vi "BinaryADR112Voltmeter.vi"() -> ()   [LabVIEW 2017]
doc: "This vi interfaces with the ADR 112 Serial Board and acts as a voltmeter, displaying the voltage as a graphical needle guage as well as a binary led array."
uses:
  <vilib>/Instr/_visa.llb/VISA Configure Serial Port (Instr).vi
panel:
  in  "Channel":i32
  in  "COM":refnum<visa-resource-name>
  in  "On":bool
  out "Voltmeter":dbl(knob) scale=0.0..5.0
  out "12 Bit Binary Display":bool[](array[boolean])
  # "Most Significant Bit"
  # "Least Significant Bit"
  # "V"
  # "Off"
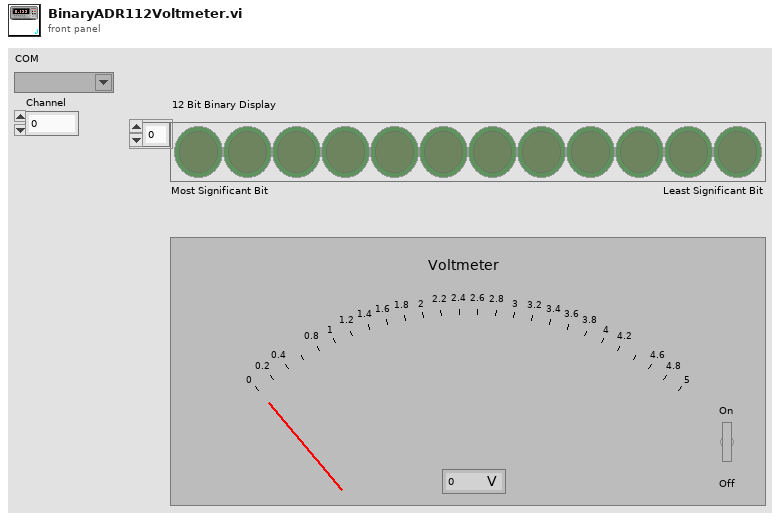
[diagram p1: front panel]
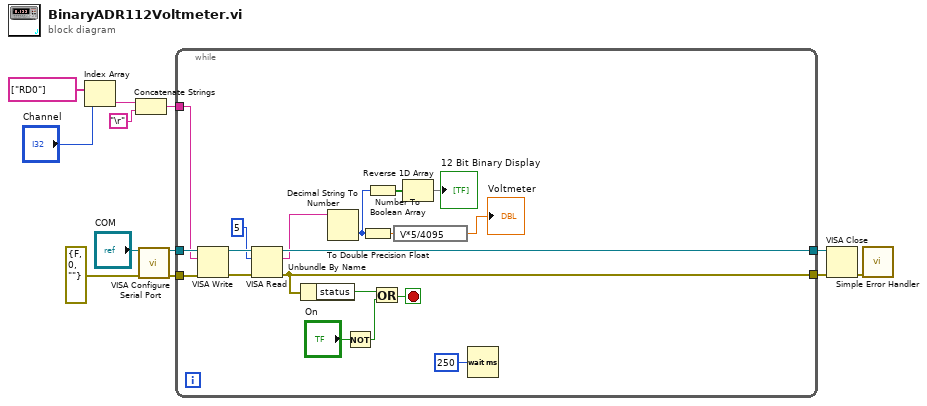
[diagram p0: block diagram]
diagram:
  n1 = Index Array(array=string[] ["RD0"], index="Channel") -> (element=w6:string)
  n2 = Concatenate Strings(w6, "\r") -> (w4:string)
  n3 = call-poly "VISA Configure Serial Port"("VISA resource name"="COM", "error in (no error)"=errorcluster {"status"=FALSE, "code"=0, "source"=""}) -> ("VISA resource name out"=w9:refnum<visa-resource-name>, "error out"=w10:errorcluster)  [unwired: 12 in]
  n4 = while {
    tunnel: w10 -> [w29]
    tunnel: w9 -> [w30]
    tunnel: w4 -> [w25]
    tunnel: [w24] -> w2
    tunnel: [w23] -> w3
    stop <- w21 stop-if-true
    n5 = VISA Write(VISA resource name=w30, write buffer=w25, error in (no error)=w29) -> (VISA resource name out=w27:refnum<visa-resource-name>, error out=w28:errorcluster)  [unwired: 1 out]
    n6 = VISA Read(VISA resource name=w27, byte count=u32 5, error in (no error)=w28) -> (VISA resource name out=w24:refnum<visa-resource-name>, read buffer=w20:string, error out=w23:errorcluster)  [unwired: 1 out]
    n7 = Unbundle By Name(w23) -> ("status"=w22:bool)
    n8 = Decimal String To Number(string=w20) -> (number=w13:i32)  [unwired: 2 in, 1 out]
    n9 = Not(x="On") -> (.not. x?=w15:bool)
    n10 = To Double Precision Float(number=w13) -> (double precision float=w19:dbl)
    n11 = Number To Boolean Array(number=w13) -> (Boolean array=w17:bool[])
    n12 = Or(x=w22, y=w15) -> (x .or. y?=w21:bool)
    n13 = expression code="V*5/4095"(w19) -> (→"Voltmeter":dbl)
    n14 = Reverse 1D Array(array=w17) -> (reversed array=→"12 Bit Binary Display":bool[])
    n15 = Wait (ms)(milliseconds to wait=u32 250) -> ()  [unwired: 1 out]
  }
  n16 = VISA Close(VISA resource name=w2, error in (no error)=w3) -> (error out=w1:errorcluster)
  n17 = call <vilib>:"Simple Error Handler.vi"("error in (no error)"=w1) -> ()  [unwired: 4 in, 5 out]
